vi "Configure Sys (To) Mode (Duty Cycle).vi"(4 "DC Off (10)":i32=10, 6 "DC On (10)":i32=10, 8 "error in (no error)":errorcluster, 9 "Period (100 msec)":dbl=0.1 format="%.6p", 11 "VISA resource name":refnum<visa-resource-name>) -> (0 "error out":errorcluster, 3 "VISA resource name out":refnum<visa-resource-name>)   [LabVIEW 2012, in "Berkeley Nucleonics 500 Series.lvlib"]
doc: "This VI is used to configure the duty cycle mode of operation of the system timer (To)."
uses:
  Berkeley Nucleonics 500 Series.lvlib
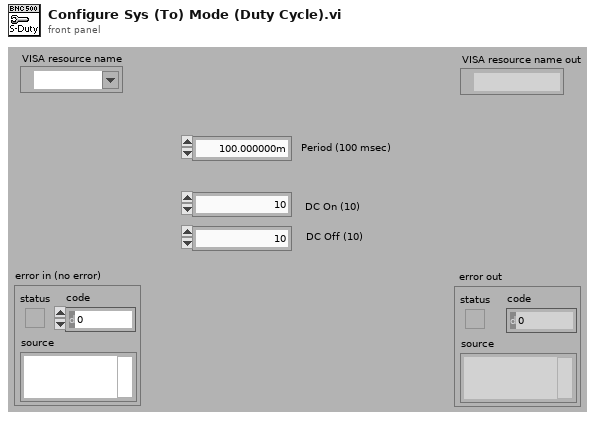
[diagram p1: front panel]
types:
  T1 = enum16{"Normal", "Single", "Burst", "Duty Cycle"}
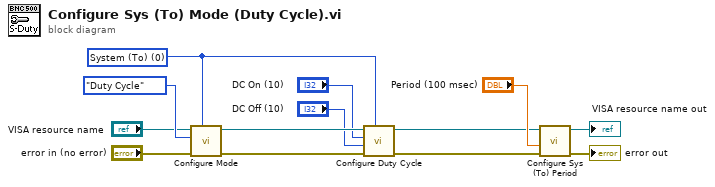
[diagram p0: block diagram]
diagram:
  w8 = 0 items=["System (To)", "Channel A", "Channel B", "Channel C", "Channel D", "Channel E", "Channel F", "Channel G", "Channel H"] ("Channel (1:Chan A)")
  n1 = call "Configure Mode.vi"("Channel (1:Chan A)"=w8, "error in (no error)"="error in (no error)", "Mode (0:Normal)"=T1."Duty Cycle" ("Chan Mode"), "VISA resource name"="VISA resource name") -> ("error out"=w12:errorcluster, "VISA resource name out"=w13:refnum<visa-resource-name>)  [unwired: 6 out]
  n2 = call "Configure Duty Cycle.vi"("Channel (1:Chan A)"=w8, "error in (no error)"=w12, "DC Off (10)"="DC Off (10)", "DC On (10)"="DC On (10)", "VISA resource name"=w13) -> ("error out"=w3:errorcluster, "VISA resource name out"=w4:refnum<visa-resource-name>)  [unwired: 5 out]
  n3 = call "Configure Sys (To) Period.vi"("error in (no error)"=w3, "Period (100 msec)"="Period (100 msec)", "VISA resource name"=w4) -> ("error out"=→"error out":errorcluster, "VISA resource name out"=→"VISA resource name out":refnum<visa-resource-name>)  [unwired: 1 in, 6 out]
